vi "NumJacobian_U.vi"(4 "Inputs":i32, 5 "F_FUNC":T1, 6 "Rows":i32, 7 "ExtraPassedData":variant, 10 "U":T2, 11 "X":T2) -> (0 "Error":bool, 3 "Result":T2)   [LabVIEW 2019, in "Trajectory_Library.lvlib"]
doc: "Returns numerical Jacobian with respect to x for f(x, u, ...).\n\nInputs: \n - rows -- Number of rows in the result of f(x, u).\n - states -- Number of rows in x.\n - f -- Vector-valued function reference from which to compute Jacobian.\n - x -- State vector.\n - u -- nput vector.\n\nOutputs:\n - result -- The numerical Jacobian with respect to x for f(x, u, ...).\n - error -- If TRUE, an error occured."
uses:
  <vilib>/Analysis/Matrix/Datatypes/RealMatrix.ctl
  CALLBACK_FUNC_TYPE.ctl
  <vilib>/Analysis/Matrix/Numeric/Subtract/Subtract - RM,RM.vi
  Trajectory_Library.lvlib
  <vilib>/Analysis/Matrix/NI_Matrix.lvlib
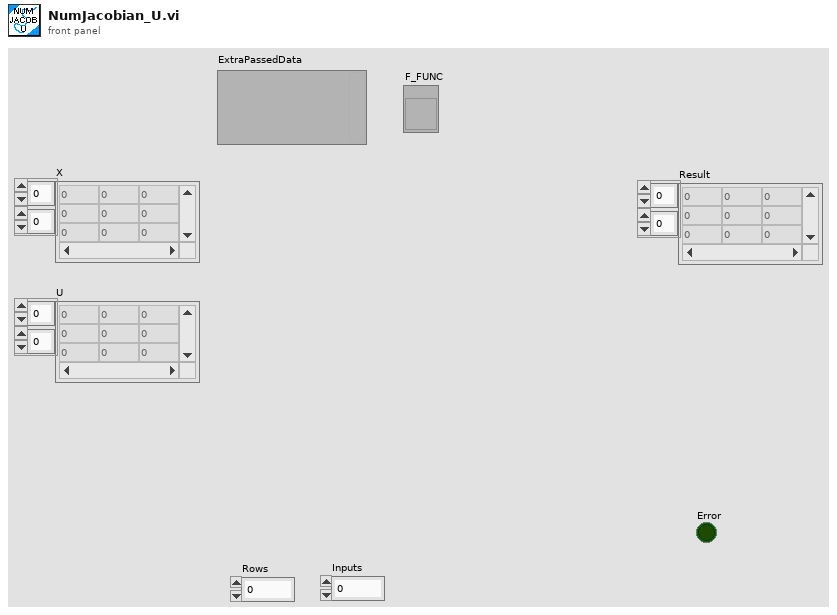
[diagram p1: front panel]
types:
  T1 = typedef "Trajectory_Library.lvlib/CALLBACK_FUNC_TYPE.ctl" = refnum<vi>
  T2 = typedef "NI_Matrix.lvlib/RealMatrix.ctl" = dbl[][]
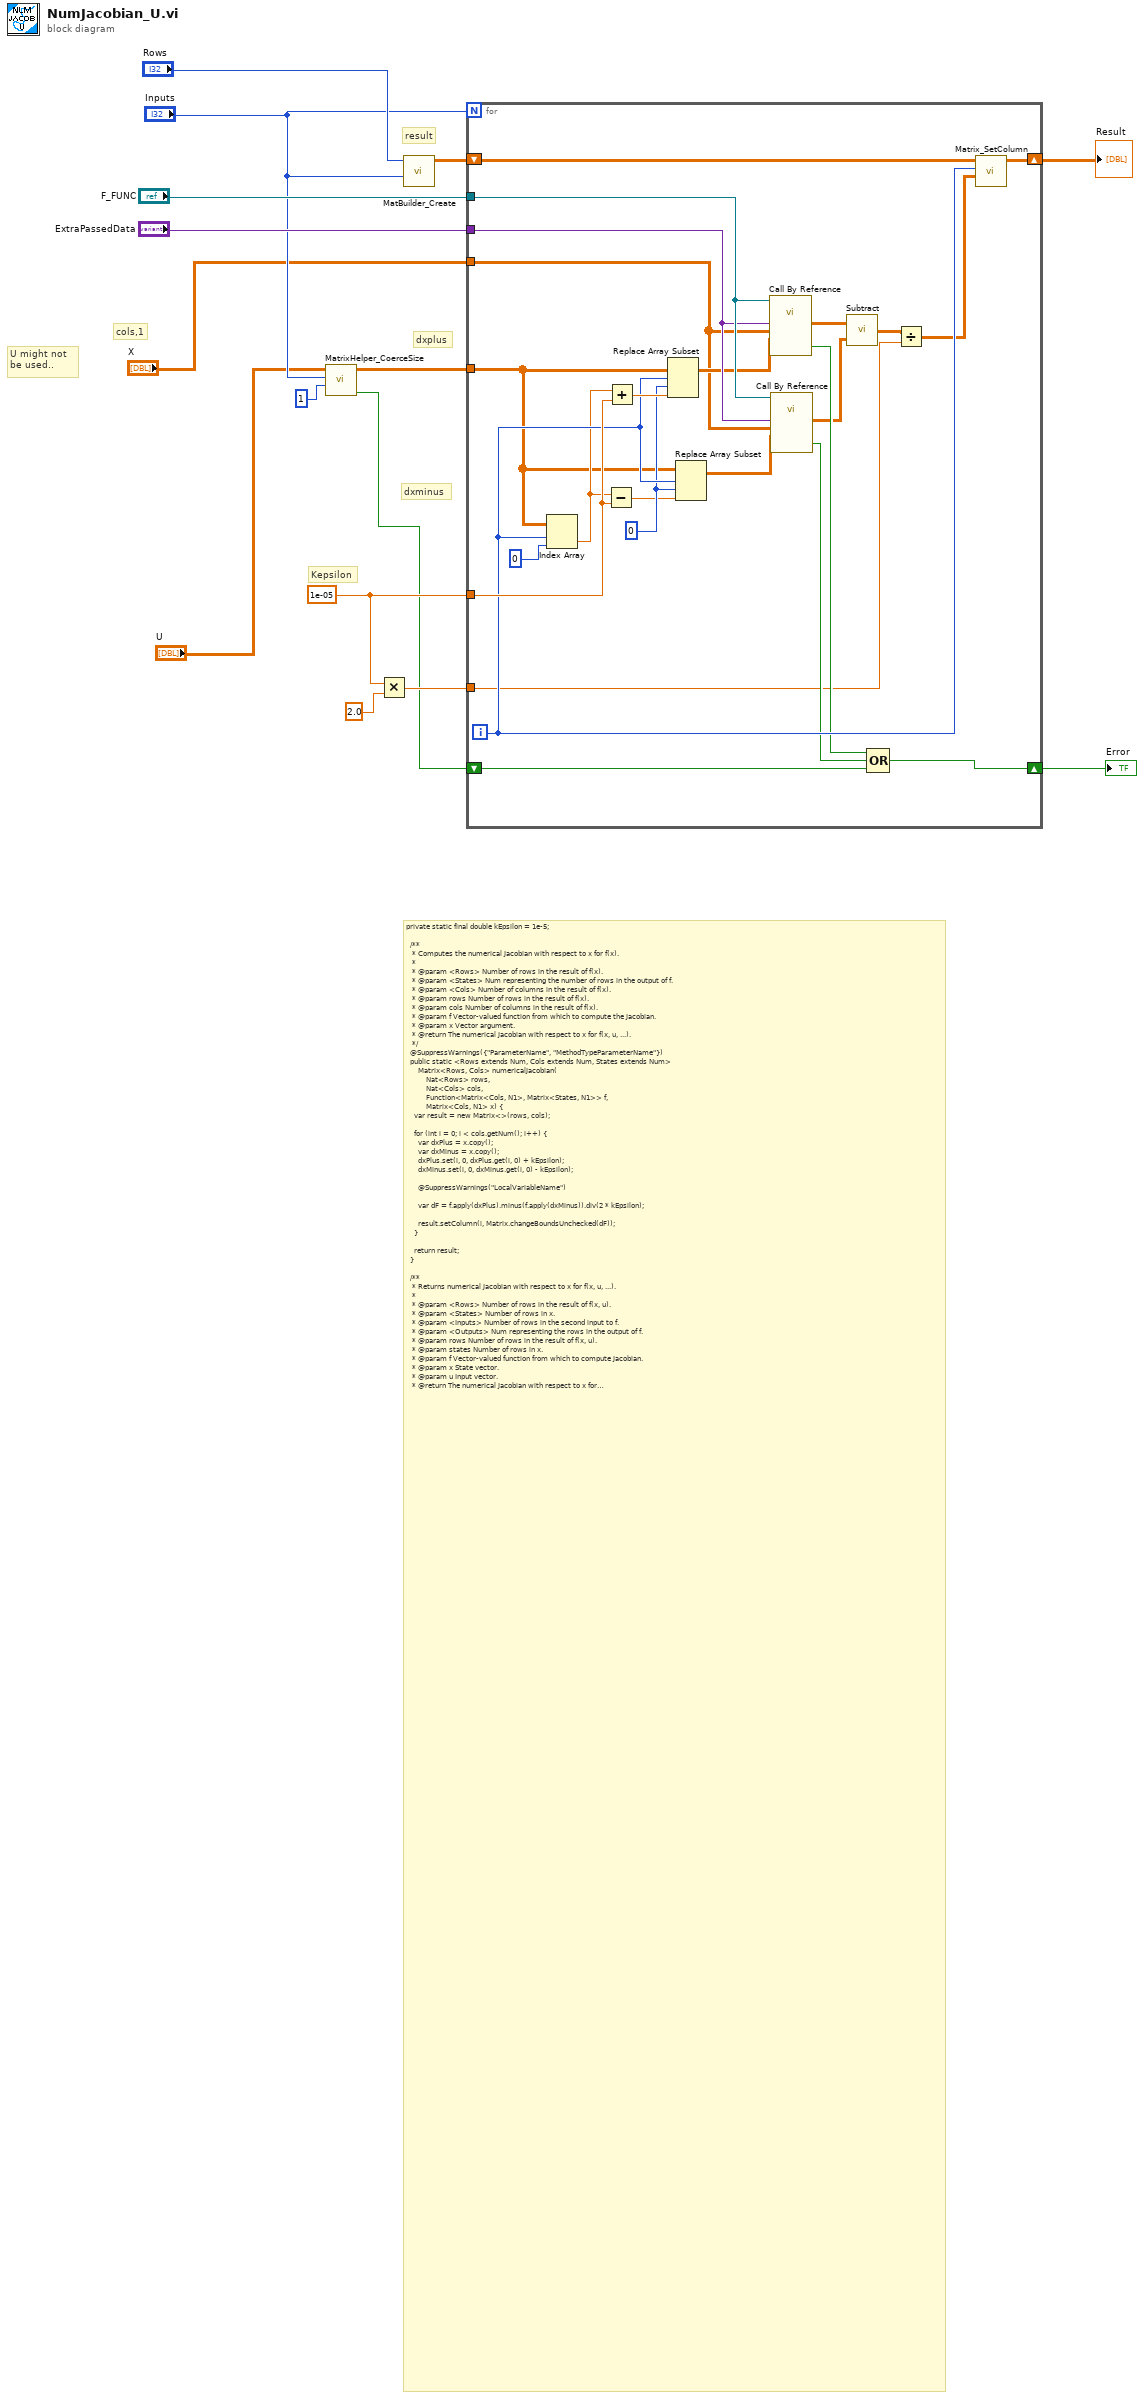
[diagram p0: block diagram]
diagram:
  w6 = 1e-05
  # "private static final double kEpsilon = 1e-5;\n\n  /**\n   * Computes the numerical Jacobian with respect to x for f(x).\n   *\n   * @param <Rows> Number of rows in the result of f(x).\n   * @param <States> Num representing the number of rows in the output of f.\n   * @param <Cols> Number of columns in the result of f(x).\n   * @param rows Number of rows in the result of f(x).\n   * @param cols Number of columns in the result of f(x).\n   * @param f Vector-valued function from which to compute the Jacobian.\n   * @param x Vector argument.\n   * @return The numerical Jacobian with respect to x for f(x, u, ...).\n   */\n  @SuppressWarnings({\"ParameterName\", \"MethodTypeParameterName\"})\n  public static <Rows extends Num, Cols extends Num, States extends Num>\n      Matrix<Rows, Cols> numericalJacobian(\n          Nat<Rows> rows,\n          Nat<Cols> cols,\n          Function<Matrix<Cols, N1>, Matrix<States, N1>> f,\n          Matrix<Cols, N1> x) {\n    var result = new Matrix<>(rows, cols);\n\n    for (int i = 0; i < cols.getNum(); i++) {\n      var dxPlus = x.copy();\n      var dxMinus = x.copy();\n      dxPlus.set(i, 0, dxPlus.get(i, 0) + kEpsilon);\n      dxMinus.set(i, 0, dxMinus.get(i, 0) - kEpsilon);\n\n      @SuppressWarnings(\"LocalVariableName\")\n\n      var dF = f.apply(dxPlus).minus(f.apply(dxMinus)).div(2 * kEpsilon);\n\n      result.setColumn(i, Matrix.changeBoundsUnchecked(dF));\n    }\n\n    return result;\n  }\n\n  /**\n   * Returns numerical Jacobian with respect to x for f(x, u, ...).\n   *\n   * @param <Rows> Number of rows in the result of f(x, u).\n   * @param <States> Number of rows in x.\n   * @param <Inputs> Number of rows in the second input to f.\n   * @param <Outputs> Num representing the rows in the output of f.\n   * @param rows Number of rows in the result of f(x, u).\n   * @param states Number of rows in x.\n   * @param f Vector-valued function from which to compute Jacobian.\n   * @param x State vector.\n   * @param u Input vector.\n   * @return The numerical Jacobian with respect to x for f(x, u, ...).\n   */\n  @SuppressWarnings({\"LambdaParameterName\", \"MethodTypeParameterName\"})\n  public static <Rows extends Num, States extends Num, Inputs extends Num, Outputs extends Num>\n      Matrix<Rows, States> numericalJacobianX(\n          Nat<Rows> rows,\n          Nat<States> states,\n          BiFunction<Matrix<States, N1>, Matrix<Inputs, N1>, Matrix<Outputs, N1>> f,\n          Matrix<States, N1> x,\n          Matrix<Inputs, N1> u) {\n    return numericalJacobian(\n                            rows, \n                            states, \n                           _x -> f.apply(_x, u), \n                            x);\n  }\n\n  /**\n   * Returns the numerical Jacobian with respect to u for f(x, u).\n   *\n   * @param <States> The states of the system.\n   * @param <Inputs> The inputs to the system.\n   * @param <Rows> Number of rows in the result of f(x, u).\n   * @param rows Number of rows in the result of f(x, u).\n   * @param inputs Number of rows in u.\n   * @param f Vector-valued function from which to compute the Jacobian.\n   * @param x State vector.\n   * @param u Input vector.\n   * @return the numerical Jacobian with respect to u for f(x, u).\n   */\n  @SuppressWarnings({\"LambdaParameterName\", \"MethodTypeParameterName\"})\n  public static <Rows extends Num, States extends Num, Inputs extends Num>\n      Matrix<Rows, Inputs> numericalJacobianU(\n          Nat<Rows> rows,\n          Nat<Inputs> inputs,\n          BiFunction<Matrix<States, N1>, Matrix<Inputs, N1>, Matrix<States, N1>> f,\n          Matrix<States, N1> x,\n          Matrix<Inputs, N1> u) {\n    return numericalJacobian(\n                rows, \n                inputs, \n                _u -> f.apply(x, _u), \n                 u);\n  }\n}"
  # "U might not \nbe used.."
  # "cols,1"
  # "dxminus"
  # "dxplus"
  # "Kepsilon"
  # "result"
  n1 = call "MatrixHelper_CoerceSize.vi"("Columns"=1, "Rows"="Inputs", "input matrix"="U") -> ("Coerced"=w3:bool, "output matrix"=w11:T2)  [unwired: 7 in]
  n2 = Multiply(x=w6, y=2.0) -> (x*y=w7:dbl)
  n3 = call "MatBuilder_Create.vi"("Columns"="Inputs", "Rows"="Rows") -> ("output matrix"=w14:T2)  [unwired: 9 in]
  n4 = for {
    N: "Inputs" -> [_]
    tunnel: w6 -> [w35]
    shift-right: [w38] -> w4
    shift-left: w14 -> [w39]
    tunnel: "F_FUNC" -> [w31]
    tunnel: "ExtraPassedData" -> [w30]
    shift-right: [w28] -> w8
    shift-left: w3 -> [w29]
    tunnel: w7 -> [w22]
    tunnel: "X" -> [w18]
    tunnel: w11 -> [w16]
    i -> [w34]
    w33 = 0 ("disabled index (col)")
    n5 = Index Array(array=w16, index (row)=w34, index (col)=0) -> (element=w17:dbl)
    n6 = Subtract(x=w17, y=w35) -> (x-y=w32:dbl)
    n7 = Add(x=w17, y=w35) -> (x+y=w36:dbl)
    n8 = Replace Array Subset(array=w16, new element=w36, index (row)=w34, index (col)=w33) -> (w20:T2)
    n9 = Replace Array Subset(array=w16, new element=w32, index (row)=w34, index (col)=w33) -> (w19:T2)
    n10 = call-by-ref "?"(reference=w31, "U"=w20, "X"=w18, "Variant"=w30) -> ("Error"=w26:bool, "NewX"=w25:T2)  [unwired: 8 in, 2 out]
    n11 = call-by-ref "?"(reference=w31, "U"=w19, "X"=w18, "Variant"=w30) -> ("Error"=w27:bool, "NewX"=w24:T2)  [unwired: 8 in, 2 out]
    n12 = call-poly <vilib>:"Subtract.vi"("Real Matrix B"=w24, "Real Matrix A"=w25) -> ("A - B"=w23:T2)
    n13 = Compound Arithmetic op=OR(w26, w27, w29) -> (w28:bool)
    n14 = Divide(x=w23, y=w22) -> (x/y=w21:T2)
    n15 = call "Matrix_SetColumn.vi"("Fill Vector"=w21, "Column"=w34, "input matrix"=w39) -> ("output matrix"=w38:T2)  [unwired: 7 in, 1 out]
  }
  "Result" <- w4
  "Error" <- w8
